vi "ProcessImagesManual.vi"() -> ()   [LabVIEW 2015]
uses:
  <vilib>/vision/Image Controls.llb/IMAQ Image.ctl
  <vilib>/vision/NI_Vision_Development_Module.lvlib
panel:
  in  "File Path":path
  out "Green":T1
  out "Copy":T1
  out "Parsed":T1
  out "Camera Image":T1(plugin-control)
  out "Targets":T1(plugin-control)
  in  "Hue Range":cluster{"Lower value":i32, "Upper value":i32}={"Lower value"=72, "Upper value"=120}
  in  "Sat Range":cluster{"Lower value":i32, "Upper value":i32}={"Lower value"=60, "Upper value"=255}
  in  "Luma Range":cluster{"Lower value":i32, "Upper value":i32}={"Lower value"=40, "Upper value"=255}
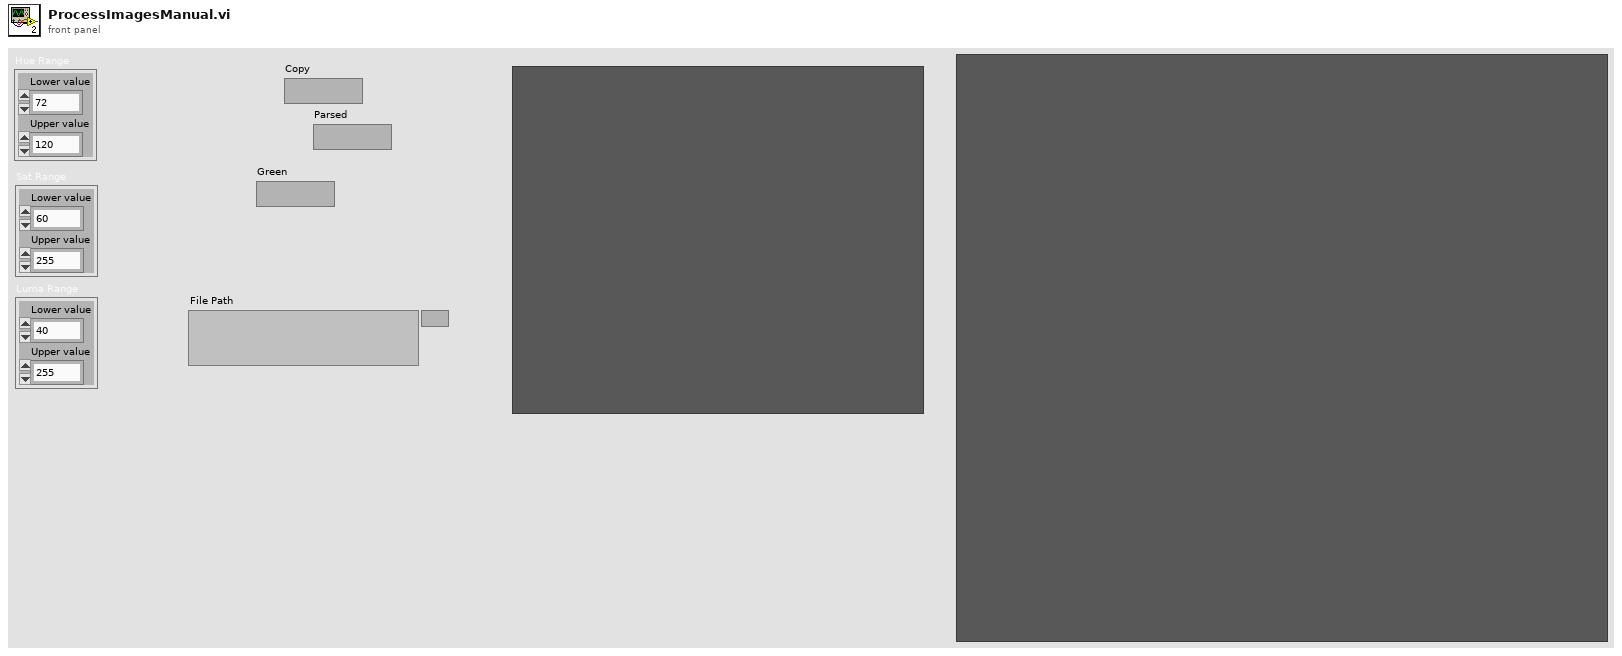
[diagram p1: front panel]
types:
  T1 = typedef "IMAQ Image.ctl" = refnum<image>
  T2 = typedef "Image Type" = u32
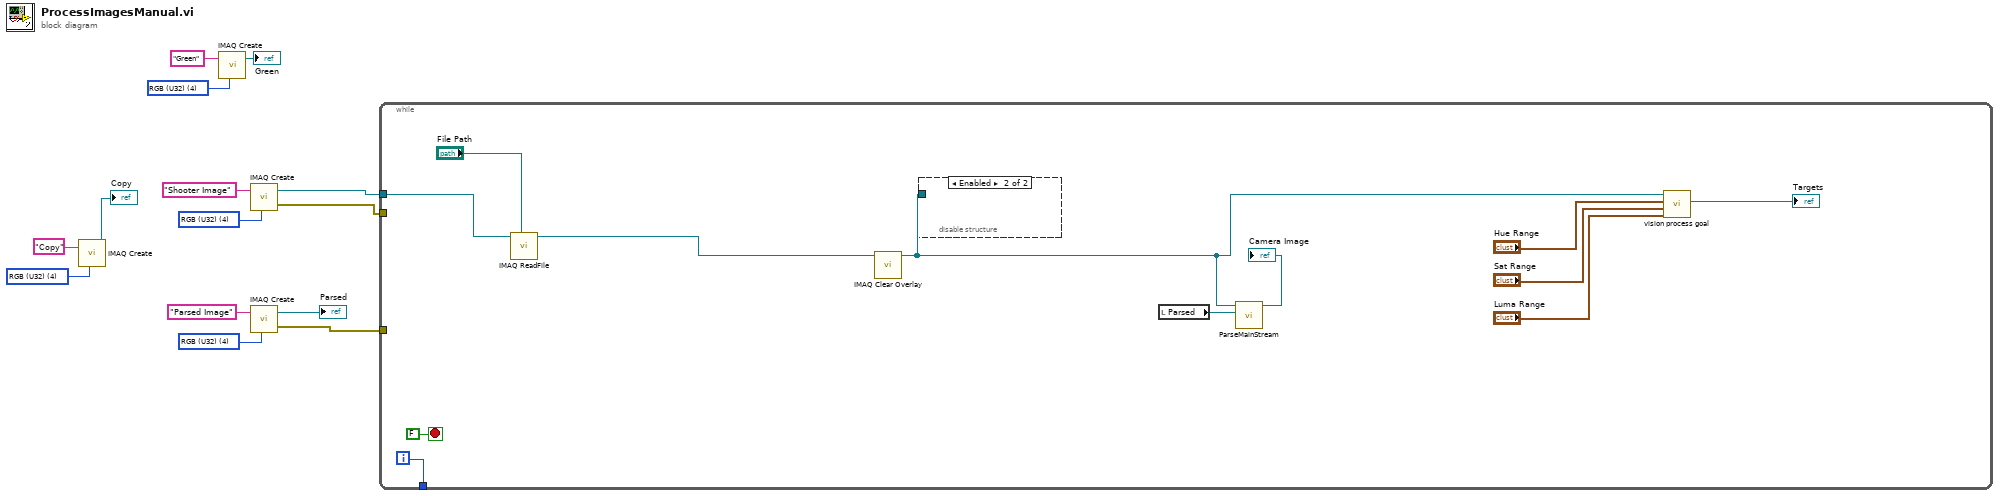
[diagram p0: block diagram]
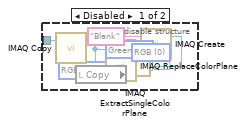
[diagram p2: hidden frame]
diagram:
  w7 = T2 4 items=["Grayscale (U8)", "Grayscale (I16)", "Grayscale (SGL)", "Complex (CSG)", "RGB (U32)", "HSL (U32)", "RGB (U64)"] ("Image Type")
  w9 = T2 4 items=["Grayscale (U8)", "Grayscale (I16)", "Grayscale (SGL)", "Complex (CSG)", "RGB (U32)", "HSL (U32)", "RGB (U64)"] ("Image Type")
  w12 = T2 4 items=["Grayscale (U8)", "Grayscale (I16)", "Grayscale (SGL)", "Complex (CSG)", "RGB (U32)", "HSL (U32)", "RGB (U64)"] ("Image Type")
  w14 = T2 4 items=["Grayscale (U8)", "Grayscale (I16)", "Grayscale (SGL)", "Complex (CSG)", "RGB (U32)", "HSL (U32)", "RGB (U64)"] ("Image Type")
  n1 = call "IMAQ Create"("Image Name"="Copy", "Image Type"=w7) -> ("New Image"=→"Copy":T1)  [unwired: 2 in, 2 out]
  n2 = call "IMAQ Create"("Image Name"="Green", "Image Type"=w9) -> ("New Image"=→"Green":T1)  [unwired: 2 in, 2 out]
  n3 = call "IMAQ Create"("Image Name"="Shooter Image", "Image Type"=w14) -> ("New Image"=w1:T1, "error out"=w2:errorcluster)  [unwired: 2 in, 1 out]
  n4 = call "IMAQ Create"("Image Name"="Parsed Image", "Image Type"=w12) -> ("New Image"=→"Parsed":T1, "error out"=w3:errorcluster)  [unwired: 2 in, 1 out]
  n5 = while {
    tunnel: [w25] -> _
    tunnel: w1 -> [w17]
    tunnel: w3 -> [_]
    tunnel: w2 -> [_]
    i -> [w25]
    stop <- FALSE stop-if-true
    n6 = call "IMAQ ReadFile"("File Path"="File Path", "Image"=w17) -> ("Image Out"=w16:T1)  [unwired: 5 in, 4 out]
    n7 = call "IMAQ Clear Overlay"("Image"=w16) -> ("Image Out"=w18:T1)  [unwired: 2 in, 8 out]
    n8 = disable-structure shown="Enabled" {
      disable-tunnel: w18 -> [w29 _]
      frame Disabled {
        w31 = 1 items=["Red", "Green", "Blue", "Hue", "Saturation", "Luminance", "Value", "Intensity"] ("Color Plane")
        w34 = T2 4 items=["Grayscale (U8)", "Grayscale (I16)", "Grayscale (SGL)", "Complex (CSG)", "RGB (U32)", "HSL (U32)", "RGB (U64)"] ("Image Type")
        w35 = u16 0 items=["RGB", "HSL", "HSV", "HSI"] ("Color Mode")
        n9 = local read "Copy"() -> (w28:T1)
        n10 = call "IMAQ Copy"("Image Dst"=w28, "Image Src"=w29) -> ("Image Dst Out"=w27:T1)  [unwired: 4 in, 1 out]
        n11 = call "IMAQ ExtractSingleColorPlane"("Color Plane"=w31, "Image Src"=w27) -> ("Image Dst Out"=w30:T1)  [unwired: 8 in, 1 out]
        n12 = call "IMAQ Create"("Image Name"="Blank", "Image Type"=w34) -> ("New Image"=w32:T1)  [unwired: 2 in, 2 out]
        n13 = call "IMAQ ReplaceColorPlane"("Image Src"=w27, "Color Mode"=w35, "Red or Hue Plane"=w32, "Green or Sat Plane"=w30, "Blue or Luma or Val or Inten Plane"=w32) -> ()  [unwired: 9 in, 2 out]
      }
      frame Enabled {
      }
    }
    n14 = local read "Parsed"() -> (w20:T1)
    n15 = call "ParseMainStream.vi"("Image Dst"=w20, "Image"=w18) -> ("Image Out"=→"Camera Image":T1)  [unwired: 9 in]
    n16 = call "vision process goal.vi"("Luma Range"="Luma Range", "Sat Range"="Sat Range", "Hue Range"="Hue Range", "Src Image"=w18) -> ("Annotated Image Out"=→"Targets":T1)  [unwired: 4 in, 3 out]
  }
